vi "NanotecSMCPDDriver.Close.vi"(0 "VISA resource name":refnum<visa-resource-name>, 1 "contollerID":i32=-1, 5 "error in (no error)":errorcluster) -> (19 "error out":errorcluster)   [LabVIEW 2014, in "NanotecSMCPDDriver.lvlib"]
doc: "Performs an instrument error query before terminating the software connection to the instrument."
uses:
  NanotecSMCPDDriver.lvlib
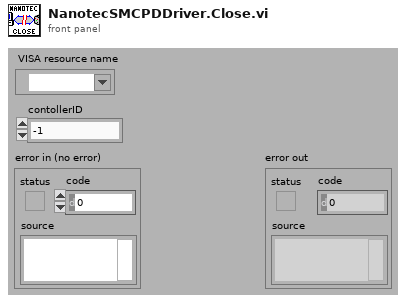
[diagram p1: front panel]
types:
  T1 = enum16{"unknown", "add", "remove", "get", "cleanup"}
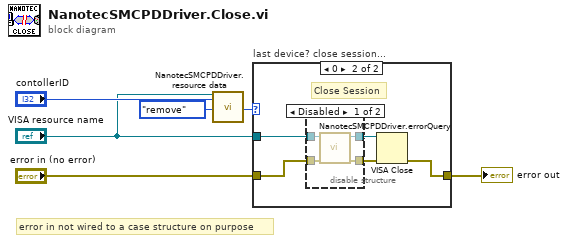
[diagram p0: block diagram]
diagram:
  # "error in not wired to a case structure on purpose"
  n1 = call "NanotecSMCPDDriver.resource data.vi"("VISAresource"="VISA resource name", "contollerID"="contollerID", "action"=T1."remove") -> ("connectionCounter"=w3:i32)  [unwired: 12 in, 4 out]
  n2 = case "last device? close session..." shown="0" w3 {
    tunnel: [w7 w12] -> w6
    tunnel: "VISA resource name" -> [_ w11]
    tunnel: "error in (no error)" -> [w7 w10]
    frame Default {
    }
    frame 0 {
      # "Close Session"
      n3 = disable-structure "Diagram Disable Structure" shown="Disabled" {
        disable-tunnel: w11 -> [w16 w18]
        disable-tunnel: w10 -> [w15 w17]
        disable-tunnel: [w14 w17] -> w9
        disable-tunnel: [w13 w18] -> w8
        frame Disabled {
          n4 = call "NanotecSMCPDDriver.errorQuery.vi"("error in (no error)"=w15, "VISA resource name"=w16) -> ("error out"=w14:errorcluster, "VISA resource name out"=w13:refnum<visa-resource-name>)  [unwired: 6 in, 2 out]
        }
        frame Enabled {
        }
      }
      n5 = VISA Close(VISA resource name=w8, error in (no error)=w9) -> (error out=w12:errorcluster)
    }
  }
  "error out" <- w6
